vi "Shut Down Device.vi"(8 "error in (no error)":errorcluster, 11 "Microscope In":refnum<class "Nikon Stand.lvclass">) -> (0 "error out":errorcluster, 3 "Microscope Out":refnum<class "Nikon Stand.lvclass">)   [LabVIEW 2023, in "Nikon Stand.lvlib" / "Nikon Stand.lvclass"]
uses:
  Nikon Stand.lvclass
  Nikon Stand.lvclass/Nikon Stand.ctl
  Microscope/ti2lv/ti2lv.lvlib
  Microscope/Microscope.lvclass
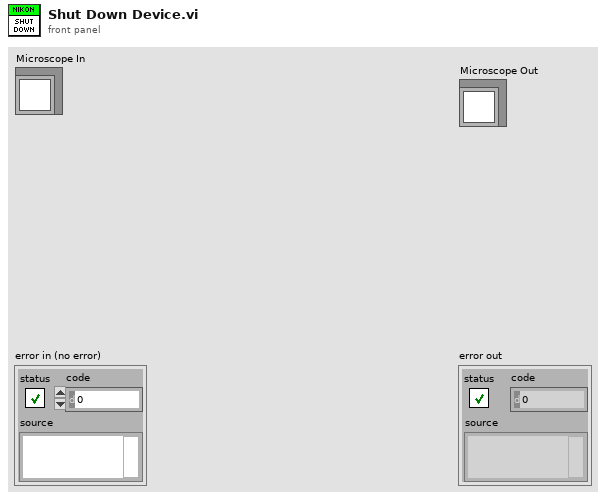
[diagram p1: front panel]
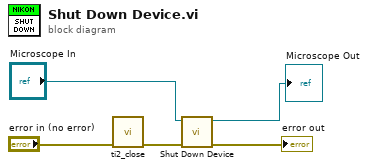
[diagram p0: block diagram]
diagram:
  n1 = call "ti2_close.vi"("error in (no error)"="error in (no error)") -> ("error out"=w3:errorcluster)  [unwired: 10 in]
  n2 = call-parent "Shut Down Device.vi"("error in (no error)"=w3, "Device in"="Microscope In") -> ("error out"=→"error out":errorcluster, "Device out"=→"Microscope Out":refnum<class "Nikon Stand.lvclass">)  [unwired: 8 in]
